vi "Smoother.vi"(8 "tolerance":dbl=0.001, 9 "B":dbl=0.97, 10 "A":dbl=0.03, 11 "Path":cluster{dbl, dbl}[](array[cluster])) -> (3 "SmoothPath":cluster{dbl, dbl}[](array[cluster]))   [LabVIEW 2018]
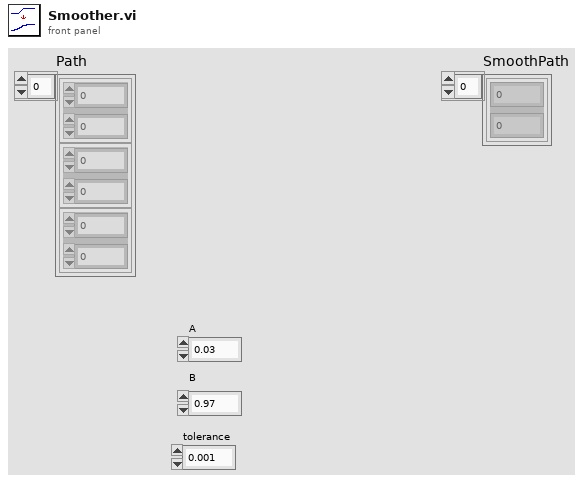
[diagram p1: front panel]
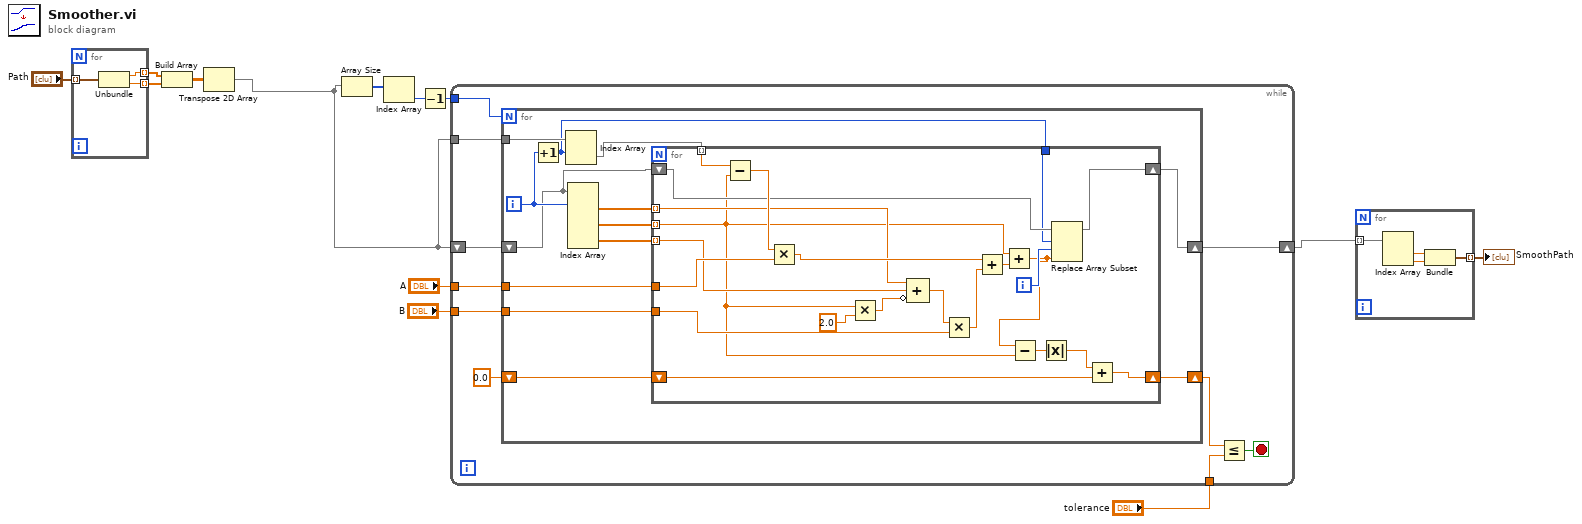
[diagram p0: block diagram]
diagram:
  n1 = for {
    tunnel: "Path" -> [w16] mode=indexing
    tunnel: [w15] -> w7 mode=indexing
    tunnel: [w14] -> w6 mode=indexing
    n2 = Unbundle(w16) -> (w15:dbl, w14:dbl)
  }
  n3 = Build Array(w7, w6) -> (w5:dbl[][])
  n4 = Transpose 2D Array(2D array=w5) -> (transposed array=w4:dbl[][])
  n5 = Array Size(array=w4) -> (size(s)=w13:i32[])
  n6 = Index Array(array=w13) -> (element=w12:i32)  [unwired: 1 in]
  n7 = Decrement(x=w12) -> (x-1=w11:i32)
  n8 = while {
    tunnel: w11 -> [w26]
    tunnel: "A" -> [w25]
    tunnel: "B" -> [w24]
    tunnel: w4 -> [w23]
    shift-right: [w21] -> w2
    shift-left: w4 -> [w22]
    tunnel: "tolerance" -> [w20]
    stop <- w19 stop-if-true
    n9 = for {
      N: w26 -> [_]
      tunnel: w25 -> [w39]
      tunnel: w24 -> [w38]
      tunnel: w23 -> [w36]
      shift-right: [w29] -> w21
      shift-left: w22 -> [w31]
      shift-right: [w28] -> w17
      shift-left: 0.0 -> [w27]
      i -> [w35]
      n10 = Increment(x=w35) -> (x+1=w30:i32)
      n11 = Index Array(array=w36, index (row)=w30) -> (element=w34:dbl[])  [unwired: 1 in]
      n12 = Index Array(array=w31, index (row) #1=w35) -> (element #1=w33:dbl[], element #2=w37:dbl[], element #3=w32:dbl[])  [unwired: 5 in]
      n13 = for {
        tunnel: w37 -> [w44] mode=indexing
        tunnel: w39 -> [w61]
        tunnel: w38 -> [w57]
        tunnel: w34 -> [w60] mode=indexing
        tunnel: w33 -> [w56] mode=indexing
        tunnel: w32 -> [w55] mode=indexing
        tunnel: w30 -> [w47]
        shift-right: [w46] -> w29
        shift-left: w31 -> [w49]
        shift-right: [w42] -> w28
        shift-left: w27 -> [w41]
        i -> [w48]
        n14 = Subtract(x=w60, y=w44) -> (x-y=w59:dbl)
        n15 = Multiply(x=w59, y=w61) -> (x*y=w58:dbl)
        n16 = Multiply(x=w44, y=2.0) -> (x*y=w54:dbl)
        n17 = Compound Arithmetic op=ADD(w56, w55, invert w54) -> (w52:dbl)
        n18 = Multiply(x=w52, y=w57) -> (x*y=w51:dbl)
        n19 = Add(x=w58, y=w51) -> (x+y=w50:dbl)
        n20 = Add(x=w44, y=w50) -> (x+y=w45:dbl)
        n21 = Subtract(x=w45, y=w44) -> (x-y=w43:dbl)
        n22 = Absolute Value(x=w43) -> (abs(x)=w40:dbl)
        n23 = Replace Array Subset(array=w49, new element=w45, index (row)=w47, index (col)=w48) -> (w46:dbl[][])
        n24 = Add(x=w40, y=w41) -> (x+y=w42:dbl)
      }
    }
    n25 = Less Or Equal?(x=w17, y=w20) -> (x <= y?=w19:bool)
  }
  n26 = for {
    tunnel: w2 -> [w65] mode=indexing
    tunnel: [w62] -> w1 mode=indexing
    n27 = Index Array(array=w65) -> (element #1=w64:dbl, element #2=w63:dbl)  [unwired: 2 in]
    n28 = Bundle(w64, w63) -> (w62:cluster{dbl, dbl})  [unwired: 1 in]
  }
  "SmoothPath" <- w1
